vi "Message from Segments.vi"(8 "error in (no error)":errorcluster, 9 "Segments in":T1[](array[typedef]), 10 "Messages in":map{string, T3}(c390), 11 "ProtoParser in":refnum<class "ProtoParser.lvclass">) -> (0 "error out":errorcluster, 1 "Remaining":T1[](array[typedef]), 2 "Messages":map{string, T3}(c390), 3 "ProtoParser out":refnum<class "ProtoParser.lvclass">)   [LabVIEW 2020, in "LV-Protoc.lvlib" / "ProtoParser.lvclass"]
uses:
  ProtoParser.lvclass
  Raw Segment.ctl
  Segment Type.ctl
  LV-Proto/Message.ctl
  LV-Proto/Field.ctl
  LV-Proto/Type.ctl
  LV-Proto/Proto Type.ctl
  LV-Proto/LV-Proto.lvlib
  LV-Protoc.lvlib
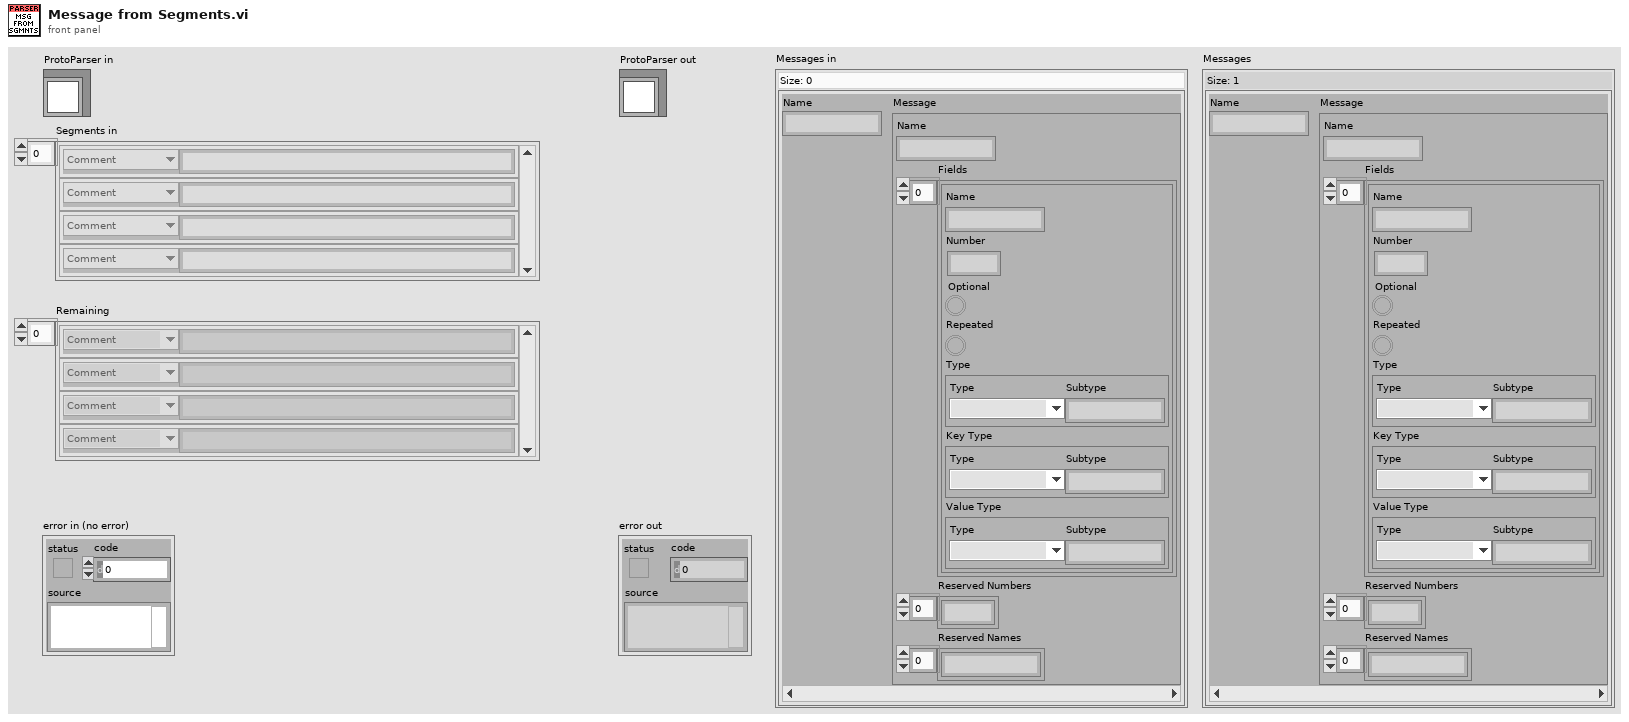
[diagram p1: front panel]
types:
  T1 = typedef "LV-Protoc.lvlib/Raw Segment.ctl" = cluster{"Type":T2, "Text":string}
  T2 = typedef "LV-Protoc.lvlib/Segment Type.ctl" = enum16{"Comment", "Message Open", "Enum Open", "Message Close", "Enum Close", "Field", "Syntax", "Import", "Enum Value", "Package", "Reserved"}
  T3 = typedef "LV-Proto.lvlib/Message.ctl" = cluster{"Name":string, "Fields":T4[], "Reserved Numbers":u32[], "Reserved Names":string[]}
  T4 = typedef "LV-Proto.lvlib/Field.ctl" = cluster{"Name":string, "Number":u32, "Optional":bool, "Repeated":bool, "Type":T5, "Key Type":T5, "Value Type":T5}
  T5 = typedef "LV-Proto.lvlib/Type.ctl" = cluster{"Type":T6, "Subtype":string}
  T6 = typedef "LV-Proto.lvlib/Proto Type.ctl" = enum16{"UNKNOWN", "double", "float", "int32", "int64", "uint32", "uint64", "sint32", "sint64", "fixed32", "fixed64", "sfixed32", "sfixed64", "bool", "string", "bytes", "enum", "map", "message"}
  T7 = typedef "LV-Protoc.lvlib/Reserved Type.ctl" = enum16{"Numeric", "Name"}
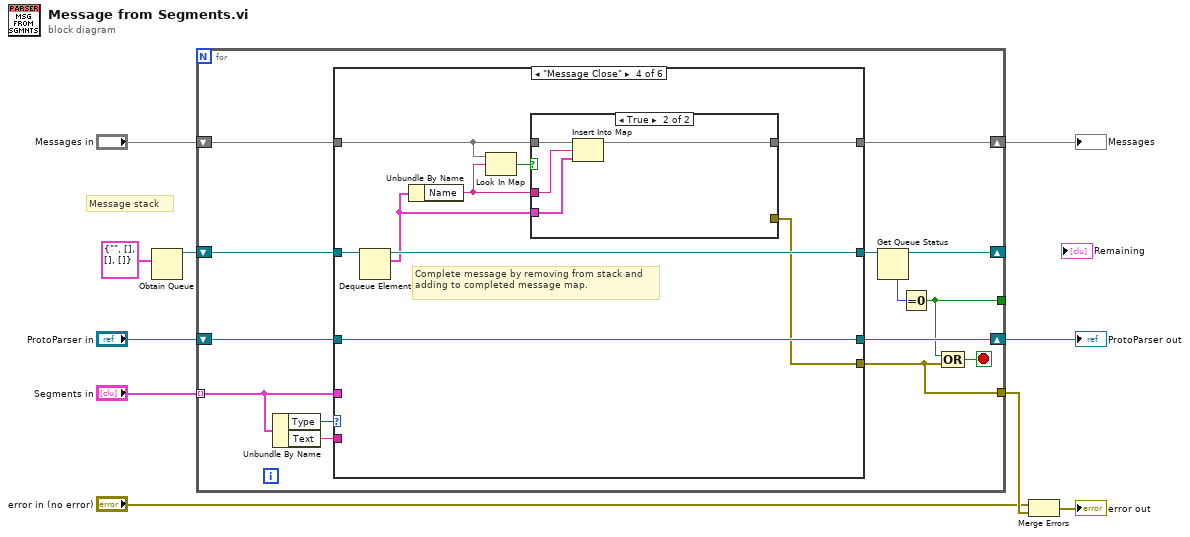
[diagram p0: block diagram]
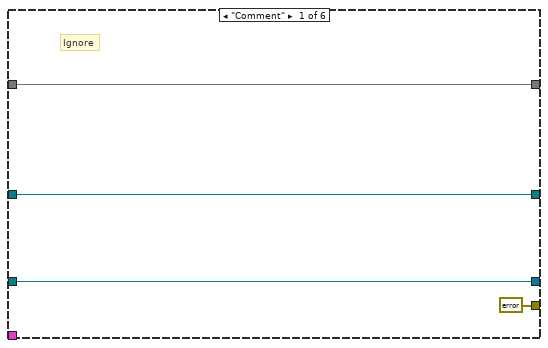
[diagram p2: hidden frame]
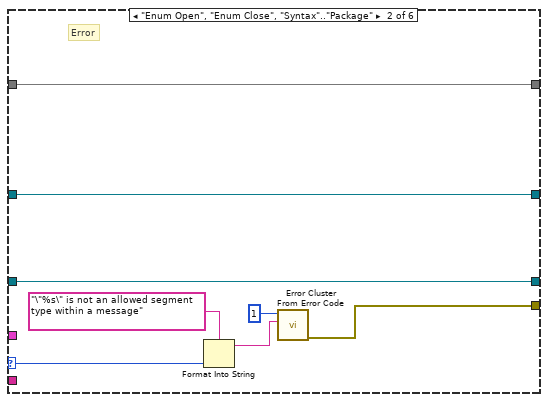
[diagram p3: hidden frame]
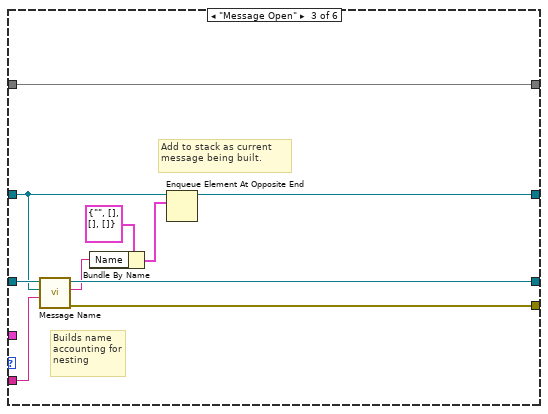
[diagram p4: hidden frame]
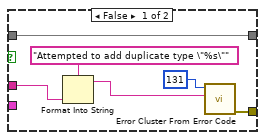
[diagram p5: hidden frame]
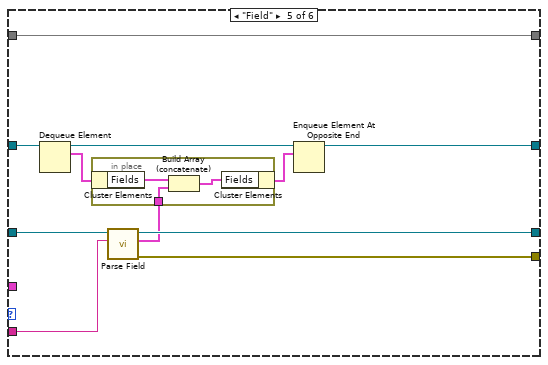
[diagram p6: hidden frame]
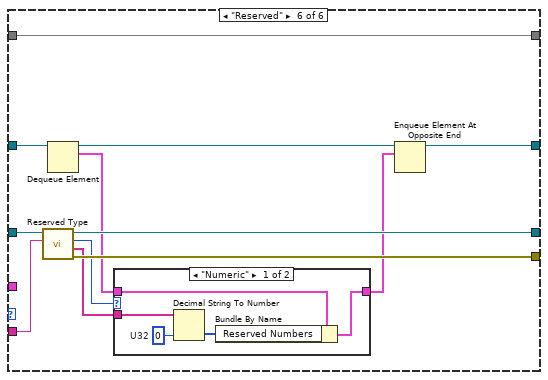
[diagram p7: hidden frame]
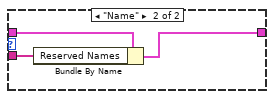
[diagram p8: hidden frame]
diagram:
  # "Message stack"
  n1 = Obtain Queue(element data type=T3 {"Name"="", "Fields"=[], "Reserved Numbers"=[], "Reserved Names"=[]} ("Message")) -> (queue out=w5:refnum<queue>)  [unwired: 4 in, 2 out]
  n2 = for {
    tunnel: "Segments in" -> [w12] mode=indexing
    shift-right: [w20] -> w10
    shift-left: "ProtoParser in" -> [w21]
    shift-right: [w15] -> _
    shift-left: w5 -> [w18]
    shift-right: [w16] -> w7
    shift-left: "Messages in" -> [w19]
    tunnel: [w13] -> _
    tunnel: [w24] -> w3
    stop <- w11 stop-if-true
    n3 = Unbundle By Name(w12) -> ("Type"=w23:T2, "Text"=w22:string)
    n4 = case shown="\"Message Close\"" w23 {
      selector: w23 -> [_ w31 _ _ _ _]
      tunnel: w22 -> [_ _ w42 _ w72 w87]
      tunnel: w12 -> [_ _ _ _ _ _]
      tunnel: w21 -> [w28 w36 w46 w55 w76 w90]
      tunnel: [w28 w36 w44 w55 w73 w88] -> w20
      tunnel: w19 -> [w26 w34 w45 w51 w74 w89]
      tunnel: w18 -> [w27 w35 w43 w54 w75 w84]
      tunnel: [w27 w35 w39 w53 w68 w81] -> w17
      tunnel: [w26 w34 w45 w48 w74 w89] -> w16
      tunnel: [errorcluster {"status"=FALSE, "code"=0, "source"=""} ("error out") w33 w37 w47 w66 w91] -> w24
      frame "Comment" {
        # "Ignore"
      }
      frame "Enum Open", "Enum Close", "Syntax".."Package" {
        # "Error"
        n5 = Format Into String(format string="\"%s\" is not an allowed segment type within a message", w31) -> (resulting string=w30:string)  [unwired: 2 in, 1 out]
        n6 = call <vilib>:"Error Cluster From Error Code.vi"("error message (\"\")"=w30, "error code (0)"=1) -> ("error out"=w33:errorcluster)  [unwired: 7 in]
      }
      frame "Message Open" {
        # "Add to stack as current message being built."
        # "Builds name accounting for nesting"
        n7 = call "Message Name.vi"("Text"=w42, "Message Stack in"=w43, "ProtoParser in"=w46) -> ("error out"=w37:errorcluster, "Message Name"=w40:string, "ProtoParser out"=w44:refnum<class "ProtoParser.lvclass">)  [unwired: 6 in]
        n8 = Bundle By Name(cluster=T3 {"Name"="", "Fields"=[], "Reserved Numbers"=[], "Reserved Names"=[]} ("Message"), "Name"=w40) -> (w38:T3)
        n9 = Enqueue Element At Opposite End(queue=w43, element=w38) -> (queue out=w39:refnum<queue>)  [unwired: 2 in, 2 out]
      }
      frame "Message Close" {
        # "Complete message by removing from stack and adding to completed message map."
        n10 = Dequeue Element(queue=w54) -> (queue out=w53:refnum<queue>, element=w49:T3)  [unwired: 2 in, 2 out]
        n11 = Unbundle By Name(w49) -> ("Name"=w50:string)
        n12 = Look In Map(map=w51, key=w50) -> (key not found?=w52:bool)  [unwired: 1 in, 1 out]
        n13 = case shown="True" w52 {
          tunnel: w51 -> [w61 w65]
          tunnel: w50 -> [w59 w64]
          tunnel: w49 -> [_ w63]
          tunnel: [w61 w62] -> w48
          tunnel: [w56 _] -> w47
          frame False {
            n14 = Format Into String(format string="Attempted to add duplicate type \"%s\"", w59) -> (resulting string=w57:string)  [unwired: 2 in, 1 out]
            n15 = call <vilib>:"Error Cluster From Error Code.vi"("error message (\"\")"=w57, "error code (0)"=131) -> ("error out"=w56:errorcluster)  [unwired: 7 in]
          }
          frame True {
            n16 = Insert Into Map(map in=w65, key=w64, value=w63) -> (map out=w62:map{string, T3})  [unwired: 2 out]
          }
        }
      }
      frame "Field" {
        n17 = Dequeue Element(queue=w75) -> (queue out=w71:refnum<queue>, element=w70:T3)  [unwired: 2 in, 2 out]
        n18 = call "Parse Field.vi"("Text"=w72, "ProtoParser in"=w76) -> ("error out"=w66:errorcluster, "Field"=w69:T4, "ProtoParser out"=w73:refnum<class "ProtoParser.lvclass">)  [unwired: 7 in]
        n19 = in-place {
          in-place-border: w69 -> [w78]
          n20 = in-place-cluster #1(w70) -> ("Fields"=w79:T4[])
          n21 = Build Array (concatenate)(w79, w78) -> (w77:T4[])
          n22 = in-place-cluster #1("Fields"=w77) -> (w67:T3)
        }
        n23 = Enqueue Element At Opposite End(queue=w71, element=w67) -> (queue out=w68:refnum<queue>)  [unwired: 2 in, 2 out]
      }
      frame "Reserved" {
        n24 = call "Reserved Type.vi"("Text"=w87, "ProtoParser in"=w90) -> ("error out"=w91:errorcluster, "Values"=w85:string[], "Reserved Type"=w86:T7, "ProtoParser out"=w88:refnum<class "ProtoParser.lvclass">)  [unwired: 6 in]
        n25 = Dequeue Element(queue=w84) -> (queue out=w82:refnum<queue>, element=w83:T3)  [unwired: 2 in, 2 out]
        n26 = case shown="\"Numeric\"" w86 {
          tunnel: w85 -> [w96 w98]
          tunnel: w83 -> [w92 w99]
          tunnel: [w93 w97] -> w80
          frame "Numeric" {
            w94 = u32 0  # U32
            n27 = Decimal String To Number(string=w96, default (0L)=w94) -> (number=w95:u32[])  [unwired: 1 in, 1 out]
            n28 = Bundle By Name(cluster=w92, "Reserved Numbers"=w95) -> (w93:T3)
          }
          frame "Name" {
            n29 = Bundle By Name(cluster=w99, "Reserved Names"=w98) -> (w97:T3)
          }
        }
        n30 = Enqueue Element At Opposite End(queue=w82, element=w80) -> (queue out=w81:refnum<queue>)  [unwired: 2 in, 2 out]
      }
    }
    n31 = Get Queue Status(queue=w17) -> (queue out=w15:refnum<queue>, # elements in queue=w14:i32)  [unwired: 2 in, 6 out]
    n32 = Equal To 0?(x=w14) -> (x = 0?=w13:bool)
    n33 = Compound Arithmetic op=OR(w13, w24) -> (w11:bool)
  }
  "ProtoParser out" <- w10
  "Messages" <- w7
  n34 = Merge Errors("error in (no error)", w3) -> (→"error out":errorcluster)
